vi "Read PV URL.vi"(8 "error in (no error)":errorcluster, 11 "PV in":refnum<class "PV.lvclass">) -> (0 "error out":errorcluster, 2 "PV URL":string, 3 "PV out":refnum<class "PV.lvclass">)   [LabVIEW 2015, in "CS++ProcessVariables.lvlib" / "PV.lvclass"]
doc: "Read PV URL"
uses:
  PV.lvclass
  PV.lvclass/PV.ctl
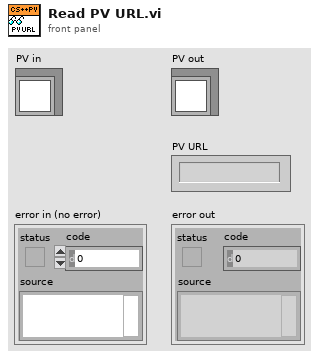
[diagram p1: front panel]
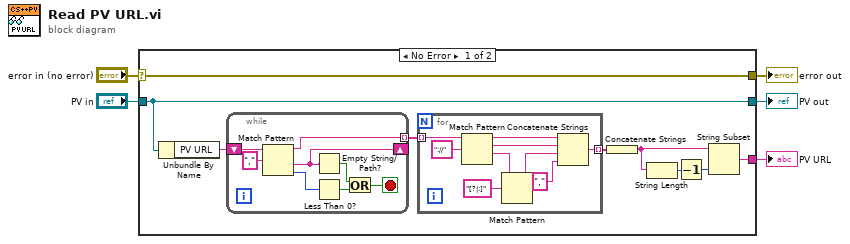
[diagram p0: block diagram]
diagram:
  n1 = case shown="No Error" "error in (no error)" {
    selector: "error in (no error)" -> [w14 w32]
    tunnel: [w14 w32] -> w4
    tunnel: [w13 w33] -> w2
    tunnel: "PV in" -> [w13 w33]
    tunnel: [w6 _] -> w1
    frame No Error {
      n2 = Unbundle By Name(w13) -> ("PV URL"=w12:string)
      n3 = while {
        shift-right: [w26] -> _
        shift-left: w12 -> [w31]
        tunnel: [w24] -> w11 mode=indexing
        stop <- w28 stop-if-true
        n4 = Match Pattern(string=w31, regular expression=",") -> (before substring=w24:string, after substring=w26:string, offset past match=w29:i32)  [unwired: 1 in, 1 out]
        n5 = Empty String/Path?(string/path=w26) -> (empty?=w25:bool)
        n6 = Less Than 0?(x=w29) -> (x < 0?=w27:bool)
        n7 = Or(x=w25, y=w27) -> (x .or. y?=w28:bool)
      }
      n8 = for {
        tunnel: [w17] -> w7 mode=indexing
        tunnel: w11 -> [w16] mode=indexing
        n9 = Match Pattern(string=w16, regular expression="://") -> (before substring=w20:string, match substring=w19:string, after substring=w21:string)  [unwired: 1 in, 1 out]
        n10 = Match Pattern(string=w21, regular expression="[?|:]") -> (before substring=w18:string)  [unwired: 1 in, 3 out]
        n11 = Concatenate Strings(w20, w19, w18, "," ("regular expression")) -> (w17:string)
      }
      n12 = Concatenate Strings(w7) -> (w10:string)
      n13 = String Length(string=w10) -> (length=w9:i32)
      n14 = Decrement(x=w9) -> (x-1=w8:i32)
      n15 = String Subset(string=w10, length (rest)=w8) -> (substring=w6:string)  [unwired: 1 in]
    }
    frame Error {
    }
  }
  "error out" <- w4
  "PV out" <- w2
  "PV URL" <- w1
